vi "Read Flow Measurements.vi"(0 "VISA resource name":refnum<visa-resource-name>, 11 "error in (no error)":errorcluster) -> (2 "Molbloc Temperature":dbl, 3 "Upstream RPT Pressure":dbl, 4 "VISA resource name out":refnum<visa-resource-name>, 6 "Ready":bool, 8 "Flow":dbl, 10 "Average Upstream Downstream RPTs":dbl, 14 "Downstream RPT Pressure":dbl, 15 "error out":errorcluster)   [LabVIEW 2023, in "Fluke Molbox 1 Plus.lvlib"]
doc: "Read the next ready/not ready indication, measurement of molbloc flow, the molbox1+ upstream and downstream RPT pressure values and the molbloc temperature. \n\n<B>Note:</B>\nThe next available measurements are replied. This can take up to 1 second since the molbox1+ waits for the next flow measurement before replying."
uses:
  Fluke Molbox 1 Plus.lvlib
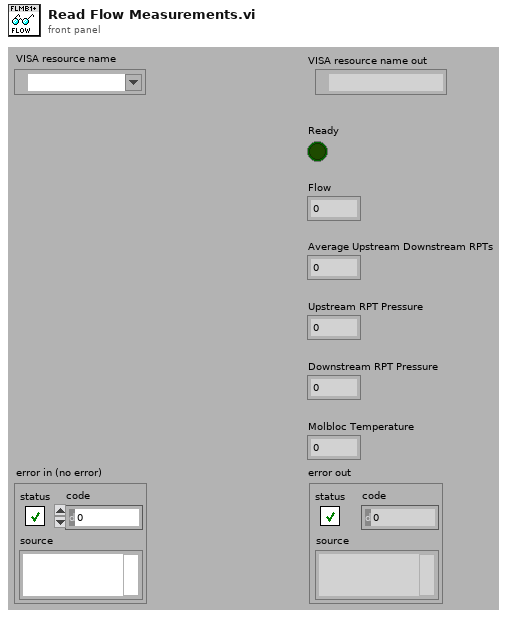
[diagram p1: front panel]
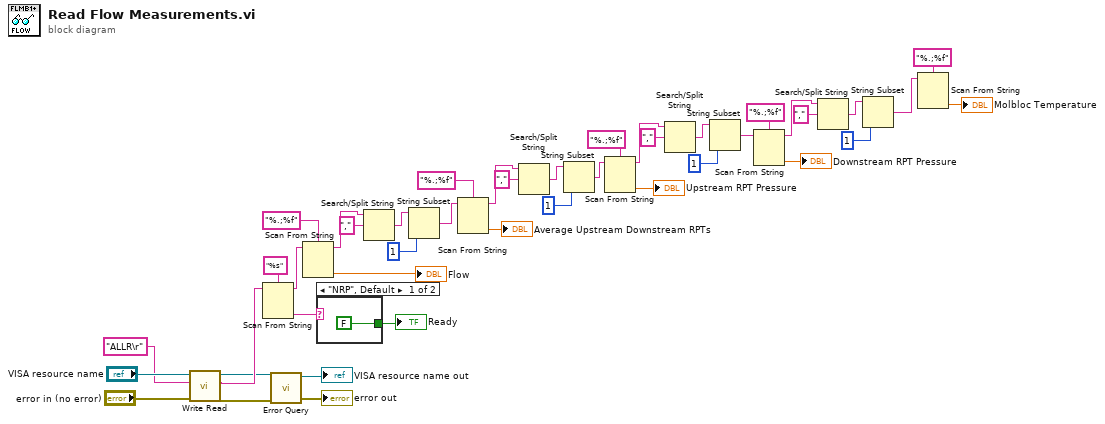
[diagram p0: block diagram]
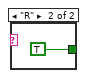
[diagram p2: hidden frame]
diagram:
  n1 = call "Write Read.vi"("error in (no error)"="error in (no error)", "Write String"="ALLR\r" ("write buffer"), "VISA resource name"="VISA resource name") -> ("error out"=w2:errorcluster, "Read Response"=w5:string, "VISA resource name out"=w1:refnum<visa-resource-name>)  [unwired: 6 in]
  n2 = Scan From String(format string="%s", input string=w5) -> (remaining string=w33:string, output 1=w41:string)  [unwired: 3 in, 2 out]
  n3 = call "Error Query.vi"("error in (no error)"=w2, "VISA resource name"=w1) -> ("error out"=→"error out":errorcluster, "VISA resource name out"=→"VISA resource name out":refnum<visa-resource-name>)  [unwired: 6 in, 2 out]
  n4 = Scan From String(format string="%.;%f", input string=w33) -> (remaining string=w9:string, output 1=→"Flow":dbl)  [unwired: 3 in, 2 out]
  n5 = case shown="\"NRP\", Default" w41 {
    tunnel: [FALSE TRUE] -> w40
    frame "NRP", Default {
    }
    frame "R" {
    }
  }
  "Ready" <- w40
  n6 = Search/Split String(string=w9, search string/char (-)=",") -> (match + rest of string=w15:string)  [unwired: 1 in, 2 out]
  n7 = String Subset(string=w15, offset (0)=1) -> (substring=w13:string)  [unwired: 1 in]
  n8 = Scan From String(format string="%.;%f", input string=w13) -> (remaining string=w11:string, output 1=→"Average Upstream Downstream RPTs":dbl)  [unwired: 3 in, 2 out]
  n9 = Search/Split String(string=w11, search string/char (-)=",") -> (match + rest of string=w19:string)  [unwired: 1 in, 2 out]
  n10 = String Subset(string=w19, offset (0)=1) -> (substring=w17:string)  [unwired: 1 in]
  n11 = Scan From String(format string="%.;%f", input string=w17) -> (remaining string=w30:string, output 1=→"Upstream RPT Pressure":dbl)  [unwired: 3 in, 2 out]
  n12 = Search/Split String(string=w30, search string/char (-)=",") -> (match + rest of string=w28:string)  [unwired: 1 in, 2 out]
  n13 = String Subset(string=w28, offset (0)=1) -> (substring=w26:string)  [unwired: 1 in]
  n14 = Scan From String(format string="%.;%f", input string=w26) -> (remaining string=w22:string, output 1=→"Downstream RPT Pressure":dbl)  [unwired: 3 in, 2 out]
  n15 = Search/Split String(string=w22, search string/char (-)=",") -> (match + rest of string=w24:string)  [unwired: 1 in, 2 out]
  n16 = String Subset(string=w24, offset (0)=1) -> (substring=w21:string)  [unwired: 1 in]
  n17 = Scan From String(format string="%.;%f", input string=w21) -> (output 1=→"Molbloc Temperature":dbl)  [unwired: 3 in, 3 out]
